vi "Vision Shooting.vi"(10 "Start Vision":bool, 11 "error in (no error)":errorcluster) -> (3 "error out":errorcluster)   [LabVIEW 2015]
uses:
  Robot Global Data.vi
panel:
  in  "Keep Vision Running":bool
  in  "Vision Running":bool
  out "What to do 2nd":string
  out "What to do 1st":string
  in  "Time In":dbl=0.25
  in  "Speed In":dbl=0.14
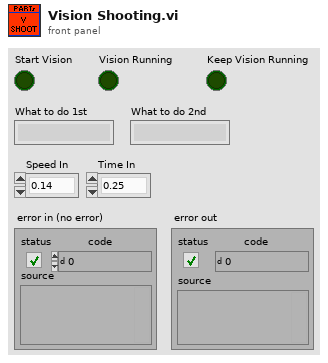
[diagram p1: front panel]
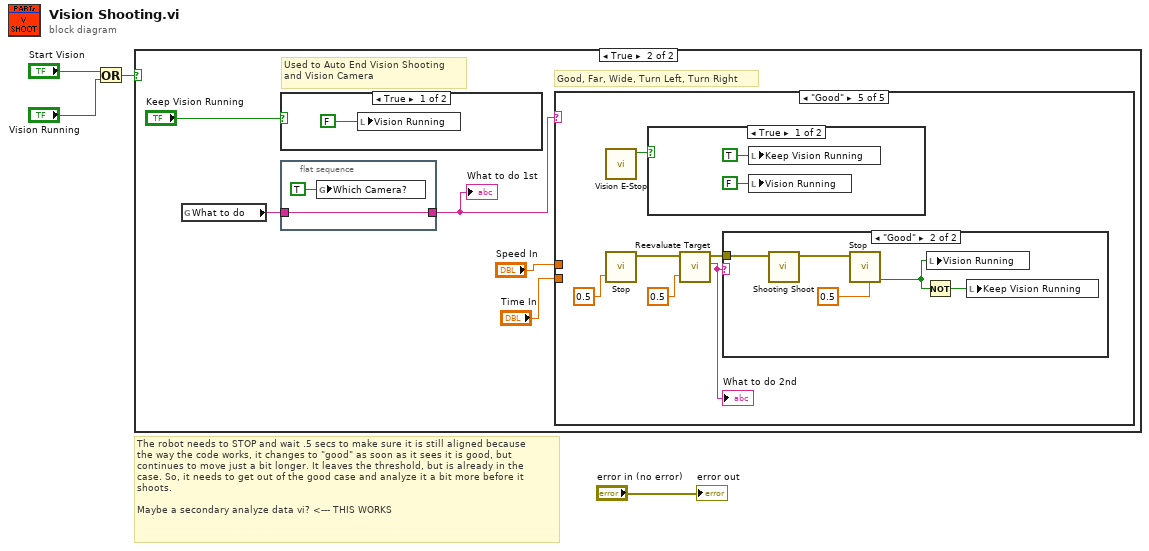
[diagram p0: block diagram]
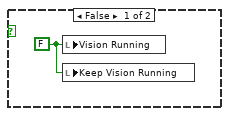
[diagram p2: hidden frame]
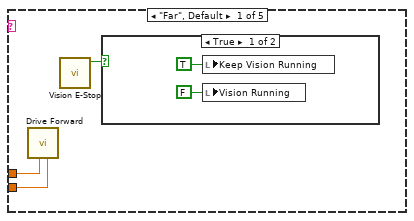
[diagram p3: hidden frame]
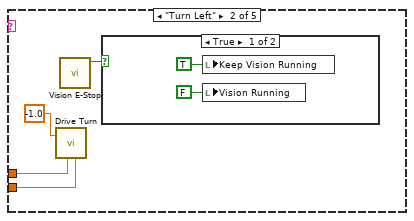
[diagram p5: hidden frame]
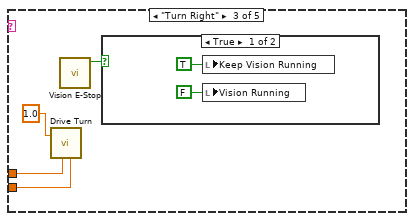
[diagram p7: hidden frame]
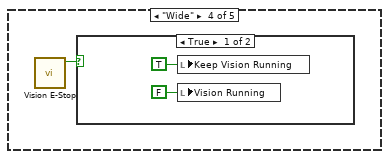
[diagram p9: hidden frame]
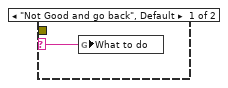
[diagram p12: hidden frame]
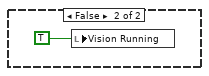
[diagram p13: hidden frame]
diagram:
  # "The robot needs to STOP and wait .5 secs to make sure it is still aligned because \nthe way the code works, it changes to \"good\" as soon as it sees it is good, but \ncontinues to move just a bit longer. It leaves the threshold, but is already in the \ncase. So, it needs to get out of the good case and analyze it a bit more before it \nshoots.\n\nMaybe a secondary analyze data vi? <--- THIS WORKS"
  n1 = Or(x="Start Vision", y="Vision Running") -> (x .or. y?=w3:bool)
  n2 = case shown="True" w3 {
    frame False {
      w5 = FALSE ("Vision Running")
      n3 = local write "Vision Running"(w5) -> ()
      n4 = local write "Keep Vision Running"(w5) -> ()
    }
    frame True {
      # "Good, Far, Wide, Turn Left, Turn Right"
      # "Used to Auto End Vision Shooting \nand Vision Camera"
      n5 = global read "Robot Global Data.vi" "What to do"() -> (w7:string)
      n6 = case shown="True" "Keep Vision Running" {
        frame True {
          n7 = local write "Vision Running"(FALSE ("Done")) -> ()
        }
        frame False {
          n8 = local write "Vision Running"(TRUE ("Done")) -> ()
        }
      }
      n9 = flat-sequence {
        tunnel: [w45] -> w6
        tunnel: w7 -> [w45]
        frame #0 {
          n10 = global write "Robot Global Data.vi" "Which Camera?"(TRUE ("Which Camera?")) -> ()
        }
      }
      n11 = case shown="\"Good\"" w6 {
        tunnel: "Speed In" -> [w13 w18 w24 _ _]
        tunnel: "Time In" -> [w12 w17 w23 _ _]
        frame "Far", Default {
          n12 = call "Drive Forward.vi"("Time"=w12, "Speed"=w13) -> ()  [unwired: 9 in, 1 out]
          n13 = call "Vision E-Stop.vi"() -> ("E-Stop"=w11:bool)  [unwired: 11 in]
          n14 = case shown="True" w11 {
            frame True {
              n15 = local write "Keep Vision Running"(TRUE ("Done")) -> ()
              n16 = local write "Vision Running"(FALSE ("Done")) -> ()
            }
            frame False {
            }
          }
        }
        frame "Turn Left" {
          n17 = call "Drive Turn.vi"("Time"=w17, "Speed"=w18, "Direction"=-1.0) -> ()  [unwired: 8 in, 1 out]
          n18 = call "Vision E-Stop.vi"() -> ("E-Stop"=w19:bool)  [unwired: 11 in]
          n19 = case shown="True" w19 {
            frame True {
              n20 = local write "Keep Vision Running"(TRUE ("Done")) -> ()
              n21 = local write "Vision Running"(FALSE ("Done")) -> ()
            }
            frame False {
            }
          }
        }
        frame "Turn Right" {
          n22 = call "Drive Turn.vi"("Time"=w23, "Speed"=w24, "Direction"=1.0) -> ()  [unwired: 8 in, 1 out]
          n23 = call "Vision E-Stop.vi"() -> ("E-Stop"=w25:bool)  [unwired: 11 in]
          n24 = case shown="True" w25 {
            frame True {
              n25 = local write "Keep Vision Running"(TRUE ("Done")) -> ()
              n26 = local write "Vision Running"(FALSE ("Done")) -> ()
            }
            frame False {
            }
          }
        }
        frame "Wide" {
          n27 = call "Vision E-Stop.vi"() -> ("E-Stop"=w28:bool)  [unwired: 11 in]
          n28 = case shown="True" w28 {
            frame True {
              n29 = local write "Keep Vision Running"(TRUE ("Done")) -> ()
              n30 = local write "Vision Running"(FALSE ("Done")) -> ()
            }
            frame False {
            }
          }
        }
        frame "Good" {
          n31 = call "Vision E-Stop.vi"() -> ("E-Stop"=w31:bool)  [unwired: 11 in]
          n32 = call "Stop.vi"("Time"=0.5) -> ("error out"=w35:errorcluster)  [unwired: 9 in, 1 out]
          n33 = case shown="True" w31 {
            frame True {
              n34 = local write "Keep Vision Running"(TRUE ("Done")) -> ()
              n35 = local write "Vision Running"(FALSE ("Done")) -> ()
            }
            frame False {
            }
          }
          n36 = call "Reevaluate Target.vi"("Delay Time (s)"=0.5 ("Time"), "error in (no error)"=w35) -> ("What to do"=w32:string, "error out (no error)"=w33:errorcluster)  [unwired: 8 in]
          "What to do 2nd" <- w32
          n37 = case shown="\"Good\"" w32 {
            selector: w32 -> [w39 _]
            tunnel: w33 -> [_ w44]
            frame "Not Good and go back", Default {
              n38 = global write "Robot Global Data.vi" "What to do"(w39) -> ()
            }
            frame "Good" {
              n39 = call "Shooting Shoot.vi"("error in (no error)"=w44) -> ("error out"=w42:errorcluster)  [unwired: 10 in]
              n40 = call "Stop.vi"("Time"=0.5, "error in"=w42) -> ("Done"=w40:bool)  [unwired: 8 in, 1 out]
              n41 = Not(x=w40) -> (.not. x?=w41:bool)
              n42 = local write "Vision Running"(w40) -> ()
              n43 = local write "Keep Vision Running"(w41) -> ()
            }
          }
        }
      }
      "What to do 1st" <- w6
    }
  }
  "error out" <- "error in (no error)"
